vi "BLE_Get_ServicesUUIDs_Property.vi"(0 ".NET Refnum in":refnum<k24>, 11 "error in (no error)":errorcluster) -> (4 ".NET Refnum out":refnum<k24>, 8 "Char Val-Property":string[][](array[string]), 15 "error out":errorcluster)   [LabVIEW 2019]
uses:
  C:/Users/chrismadlax/Desktop/LabVIEW-BLE-Driver/BLELib.dll
  BLELib.dll
panel:
  out "x-y":u32
  # "Exception"
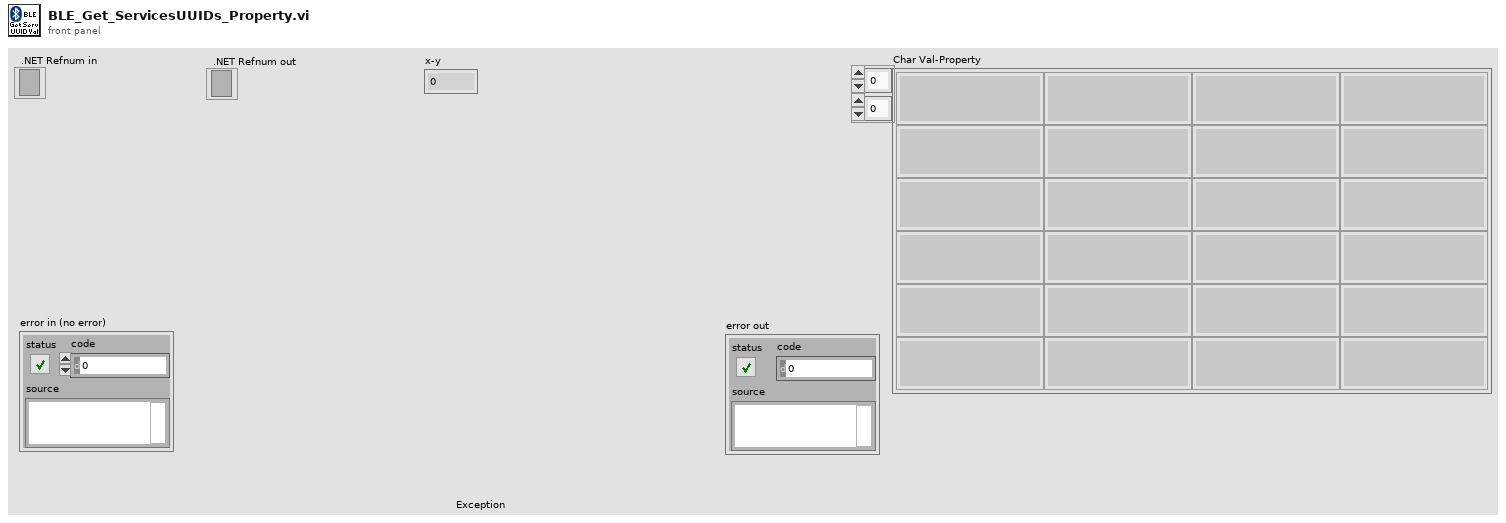
[diagram p1: front panel]
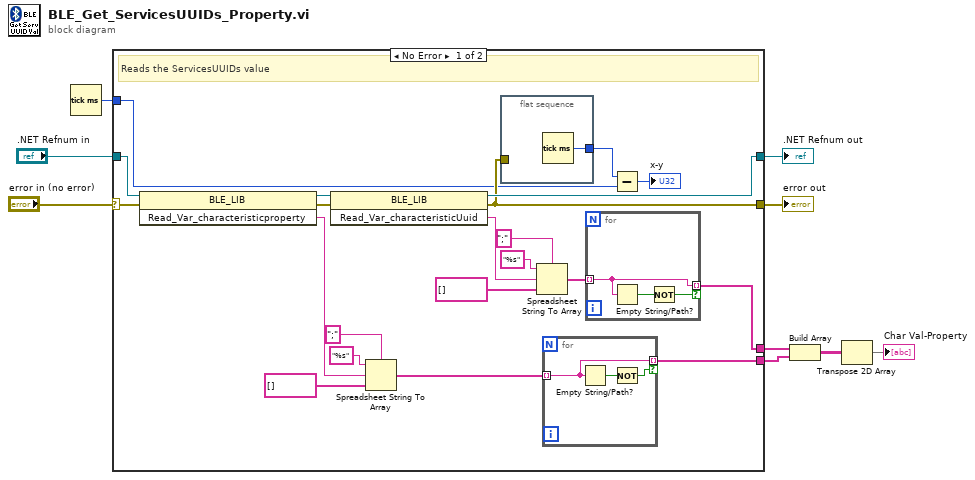
[diagram p0: block diagram]
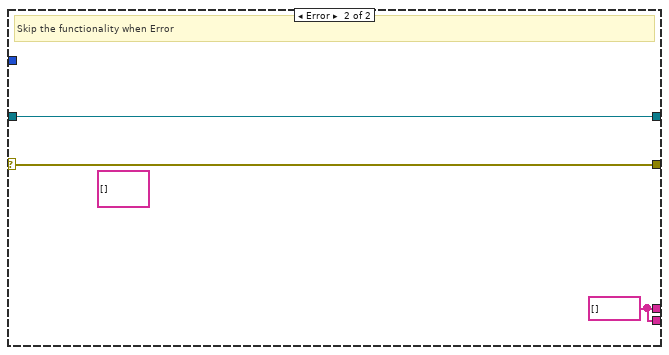
[diagram p2: hidden frame]
diagram:
  n1 = Tick Count (ms)() -> (millisecond timer value=w1:u32)
  n2 = case shown="No Error" "error in (no error)" {
    selector: "error in (no error)" -> [w11 w39]
    tunnel: ".NET Refnum in" -> [w10 w40]
    tunnel: [w15 w39] -> w8
    tunnel: [w17 w40] -> w6
    tunnel: [w25 w38] -> w4
    tunnel: [w16 w38] -> w5
    tunnel: w1 -> [w13 _]
    frame No Error {
      # "Reads the ServicesUUIDs value"
      n3 = invoke class="BLE_LIB" method="Read_Var_characteristicproperty"(reference=w10, error in=w11) -> (reference out=w19:refnum<k24>, error out=w18:errorcluster, "Read_Var_characteristicproperty"=w30:string)  [unwired: 1 in]
      n4 = invoke class="BLE_LIB" method="Read_Var_characteristicUuid"(reference=w19, error in=w18) -> (reference out=w17:refnum<k24>, error out=w15:errorcluster, "Read_Var_characteristicUuid"=w20:string)  [unwired: 1 in]
      n5 = Spreadsheet String To Array(delimiter (Tab)=";", format string="%s", spreadsheet string=w30, array type (2D Dbl)=string[] []) -> (array=w29:string[])
      n6 = flat-sequence {
        tunnel: w15 -> [_]
        tunnel: [w31] -> w14
        frame #0 {
          n7 = Tick Count (ms)() -> (millisecond timer value=w31:u32)
        }
      }
      n8 = Spreadsheet String To Array(delimiter (Tab)=";", format string="%s", spreadsheet string=w20, array type (2D Dbl)=string[] []) -> (array=w21:string[])
      n9 = for {
        tunnel: w29 -> [w37] mode=indexing
        tunnel: [w37] -> w25 mode=indexing if=w35
        n10 = Empty String/Path?(string/path=w37) -> (empty?=w36:bool)
        n11 = Not(x=w36) -> (.not. x?=w35:bool)
      }
      n12 = for {
        tunnel: w21 -> [w34] mode=indexing
        tunnel: [w34] -> w16 mode=indexing if=w32
        n13 = Empty String/Path?(string/path=w34) -> (empty?=w33:bool)
        n14 = Not(x=w33) -> (.not. x?=w32:bool)
      }
      n15 = Subtract(x=w14, y=w13) -> (x-y=→"x-y":u32)
    }
    frame Error {
      w38 = string[] []
      (unwired) string[][] []
      # "Skip the functionality when Error"
    }
  }
  "error out" <- w8
  ".NET Refnum out" <- w6
  n16 = Build Array(w5, w4) -> (w3:string[][])
  n17 = Transpose 2D Array(2D array=w3) -> (transposed array=→"Char Val-Property":string[][])
